vi "Read (Waveform)Metodo.vi"(8 "error in (no error)":errorcluster, 9 "Timeout (10000 ms)":u32=10000, 10 "Source (0: Channel 1)":u16(ring) items=["Channel 1", "Channel 2", "Channel 3", "Channel 4", "Math", "Reference A", "Reference B", "Reference C", "Reference D", "FFT"], 11 "TektroniksTDS in":refnum<class "TektroniksTDS.lvclass">) -> (0 "error out":errorcluster, 2 "Waveform Data":waveform(dbl)(graph), 3 "TektroniksTDS out":refnum<class "TektroniksTDS.lvclass">)   [LabVIEW 2020, in "TektroniksTDS.lvclass"]
uses:
  TektroniksTDS.lvclass
  TektroniksTDS.lvclass/TektroniksTDS.ctl
  <instrlib>/Tektronix TDS 200 1000 2000 Series/Tektronix TDS 200 1000 2000 Series.lvlib
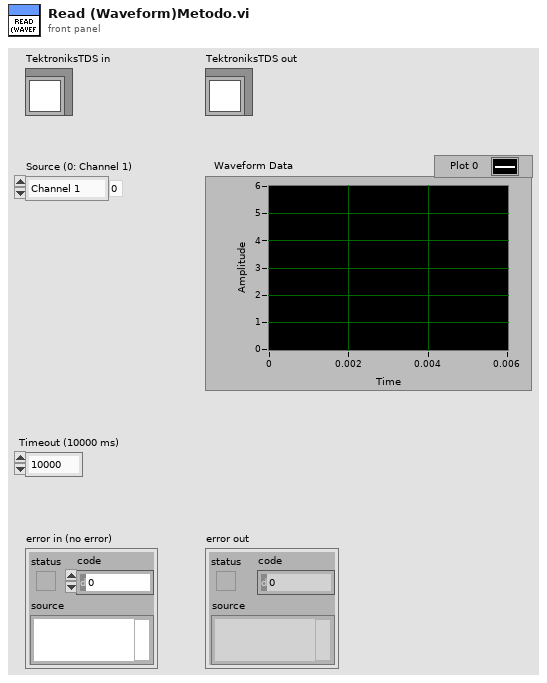
[diagram p1: front panel]
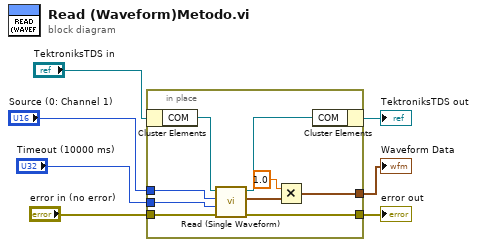
[diagram p0: block diagram]
diagram:
  n1 = in-place {
    in-place-border: [w8] -> w1
    in-place-border: [w14] -> w5
    in-place-border: "error in (no error)" -> [w13]
    in-place-border: "Source (0: Channel 1)" -> [w12]
    in-place-border: "Timeout (10000 ms)" -> [w11]
    n2 = in-place-cluster #1("TektroniksTDS in") -> ("COM"=w15:refnum<visa-resource-name>)
    n3 = call <instrlib>:"Read (Single Waveform).vi"("error in (no error)"=w13, "Timeout (10000 ms)"=w11, "Source (0: Channel 1)"=w12, "VISA resource name"=w15) -> ("error out"=w14:errorcluster, "Waveform Data"=w9:waveform(dbl), "VISA resource name out"=w16:refnum<visa-resource-name>)  [unwired: 5 in]
    n4 = Multiply(x=1.0, y=w9) -> (x*y=w8:waveform(dbl))
    n5 = in-place-cluster #1("COM"=w16) -> (→"TektroniksTDS out":refnum<class "TektroniksTDS.lvclass">)
  }
  "Waveform Data" <- w1
  "error out" <- w5
